vi "GeneradorDeDatos.vi"(9 "MANUAL":bool, 11 "Temp":dbl) -> (0 "NTC":dbl, 2 "Grados C graf":dbl, 3 "Voltaje":dbl, 4 "Grados Cent.":string="-273,150000", 5 "Grados Fare.":string="-459,670000")   [LabVIEW 2019]
doc: "Mediante el método de Stein hant- Hart, se haya una aproximación de polinomios para hallar la temperatura mediate la resistencia NTC calculada mediante un método manual o automático (Aleatorio).\nAdemás se retornan otros parámetros adicionales."
uses:
  <vilib>/numeric/Random Number (Range) DBL.vi
  <vilib>/Analysis/baseanly.llb/A x Vector.vi
  <vilib>/Analysis/baseanly.llb/Real Inverse Matrix.vi
  <vilib>/Analysis/NI_AALBase.lvlib
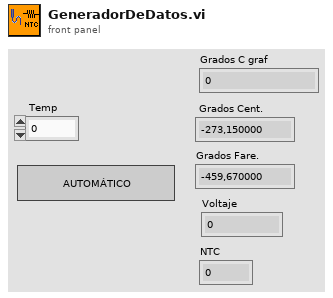
[diagram p1: front panel]
types:
  T1 = typedef "NI_Matrix.lvlib/RealMatrix.ctl" = dbl[][]
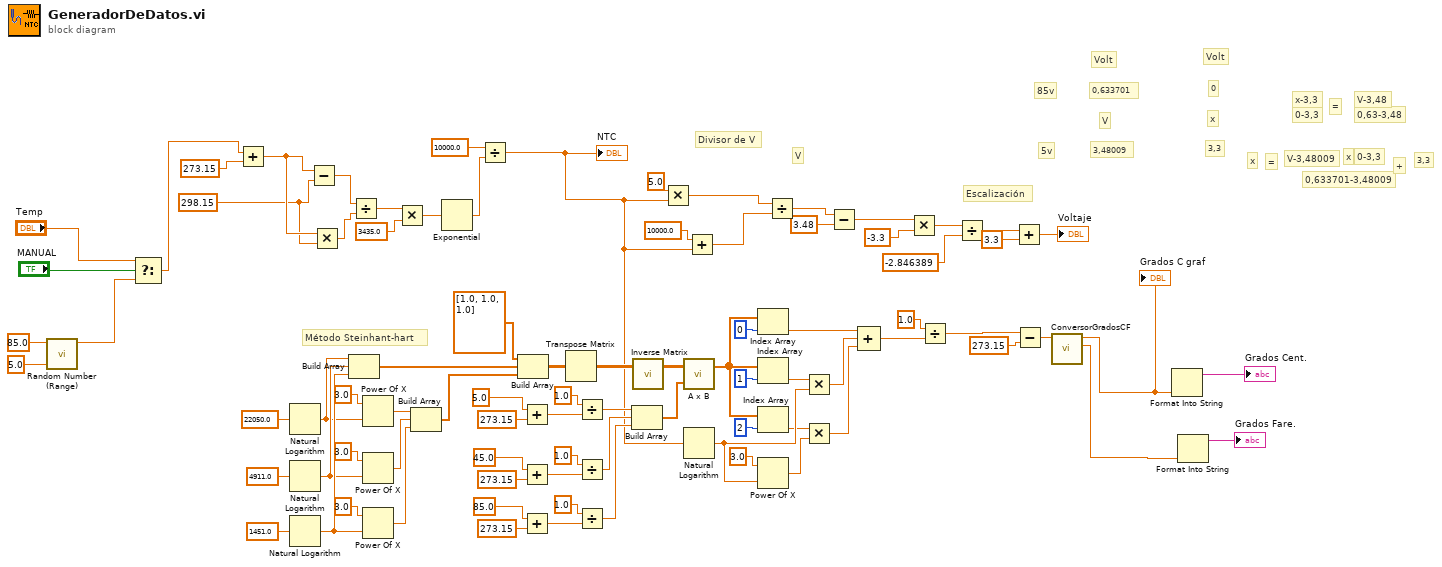
[diagram p0: block diagram]
diagram:
  w24 = 298.15 ("y")
  # "Divisor de V"
  # "V"
  # "5v"
  # "85v"
  # "="
  # "x"
  # "3,3"
  # "+"
  # "0,633701-3,48009"
  # "0-3,3"
  # "V-3,48009"
  # "x"
  # "0,63-3,48"
  # "V-3,48"
  # "="
  # "0-3,3"
  # "x-3,3"
  # "x"
  # "V"
  # "3,3"
  # "3,48009"
  # "Volt"
  # "Volt"
  # "0"
  # "0,633701"
  # "Método Steinhant-hart"
  # "Escalización"
  n1 = call-poly <vilib>:"Random Number (Range).vi"("lower bound (0)"=5.0, "upper bound (100)"=85.0) -> ("number"=w12:dbl)  [unwired: 9 in]
  n2 = Select(t="Temp", s="MANUAL", f=w12) -> (s? t:f=w11:dbl)
  n3 = Add(x=w11, y=273.15) -> (x+y=w25:dbl)
  n4 = Natural Logarithm(1:22050.0 ("y")) -> (0:w46:dbl)
  n5 = Natural Logarithm(1:4911.0 ("y")) -> (0:w47:dbl)
  n6 = Natural Logarithm(1:1451.0 ("y")) -> (0:w50:dbl)
  n7 = Subtract(x=w25, y=w24) -> (x-y=w23:dbl)
  n8 = Multiply(x=w25, y=w24) -> (x*y=w22:dbl)
  n9 = Build Array(w46, w47, w50) -> (w55:dbl[])
  n10 = Divide(x=w23, y=w22) -> (x/y=w21:dbl)
  n11 = Power Of X(1:w46, 2:3.0 ("y")) -> (0:w51:dbl)
  n12 = Power Of X(1:w47, 2:3.0 ("y")) -> (0:w52:dbl)
  n13 = Power Of X(1:w50, 2:3.0 ("y")) -> (0:w53:dbl)
  n14 = Multiply(x=w21, y=3435.0) -> (x*y=w20:dbl)
  n15 = Build Array(w51, w52, w53) -> (w56:dbl[])
  n16 = Exponential(1:w20) -> (0:w17:dbl)
  n17 = Divide(x=10000.0, y=w17) -> (x/y=w1:dbl)
  "NTC" <- w1
  n18 = Build Array(dbl[] [1.0, 1.0, 1.0], w55, w56) -> (w57:dbl[][])
  n19 = Add(x=5.0, y=273.15) -> (x+y=w30:dbl)
  n20 = Add(x=45.0, y=273.15) -> (x+y=w32:dbl)
  n21 = Add(x=85.0, y=273.15) -> (x+y=w37:dbl)
  n22 = Transpose Matrix(1:w57) -> (0:w58:dbl[][])
  n23 = Divide(x=1.0, y=w30) -> (x/y=w31:dbl)
  n24 = Divide(x=1.0, y=w32) -> (x/y=w40:dbl)
  n25 = Divide(x=1.0, y=w37) -> (x/y=w41:dbl)
  n26 = Build Array(w31, w40, w41) -> (w59:dbl[])
  n27 = call-poly <vilib>:"Inverse Matrix.vi"("Input Matrix"=w58) -> ("Inverse Matrix"=w60:T1)  [unwired: 1 in, 1 out]
  n28 = Multiply(x=5.0, y=w1) -> (x*y=w78:dbl)
  n29 = call-poly <vilib>:"A x B.vi"("Vector"=w59, "A"=w60) -> ("A x Vector"=w64:dbl[])  [unwired: 1 out]
  n30 = Natural Logarithm(1:w1) -> (0:w76:dbl)
  n31 = Add(x=10000.0 ("y"), y=w1) -> (x+y=w77:dbl)
  n32 = Index Array(array=w64, index=0) -> (element=w65:dbl)
  n33 = Index Array(array=w64, index=1) -> (element=w66:dbl)
  n34 = Index Array(array=w64, index=2) -> (element=w68:dbl)
  n35 = Power Of X(1:w76, 2:3.0 ("y")) -> (0:w69:dbl)
  n36 = Divide(x=w78, y=w77) -> (x/y=w9:dbl)
  n37 = Multiply(x=w66, y=w76) -> (x*y=w73:dbl)
  n38 = Multiply(x=w68, y=w69) -> (x*y=w70:dbl)
  n39 = Subtract(x=w9, y=3.48) -> (x-y=w7:dbl)
  n40 = Compound Arithmetic op=ADD(w65, w73, w70) -> (w72:dbl)
  n41 = Multiply(x=w7, y=-3.3) -> (x*y=w6:dbl)
  n42 = Divide(x=1.0, y=w72) -> (x/y=w75:dbl)
  n43 = Divide(x=w6, y=-2.846389) -> (x/y=w4:dbl)
  n44 = Add(x=w4, y=3.3) -> (x+y=→"Voltaje":dbl)
  n45 = Subtract(x=w75, y=273.15) -> (x-y=w81:dbl)
  n46 = call "ConversorGradosCF.vi"("GradosC"=w81) -> ("Grados F"=w85:dbl, "Grados C"=w84:dbl)  [unwired: 9 in]
  "Grados C graf" <- w84
  n47 = Format Into String "Format Into String"(w84) -> (resulting string=→"Grados Cent.":string)  [unwired: 3 in, 1 out]
  n48 = Format Into String "Format Into String"(w85) -> (resulting string=→"Grados Fare.":string)  [unwired: 3 in, 1 out]
